vi "re_Edit Remote File.vi"() -> ()   [LabVIEW 2012]
doc: "Edit a remote file by selection and downloading to a temporary file, spawning an editor, and, on completion, uploading the file back to the server when modified. This VI should be run asynchronously so as to allow for multiple editor instances. To do so, open a reference to it with the \"prepare for reentrant run\" option.\n\nBEWARE: since \"System Exec\" is used which calls into C to spawn the editor, each open editor occupies a thread. For this reason this VI has been made part of the \"Other 2\" execution system so that the threads being occupied are unlikely to be used for other tasks. Note though that as a result the number of open remote edit jobs is limited to the number of threads in the \"Other 2\" thread pool, which defaults to 4 under LabVIEW 7 with multithreading enabled."
uses:
  served/ClientSrv Server File Manipulation_srv.ctl
  typedefs/t_ClientSrv Access Levels.ctl
  glb_ClientSrv Globals.vi
panel:
  in  "Case Constant\n(See Context Help)":bool
types:
  T1 = typedef "t_ClientSrv Access Levels.ctl" = enum16{"observer", "operator", "local"}
  T2 = typedef "ClientSrv Server File Manipulation_srv.ctl" = refnum<vi>
  T3 = enum32{"existing file", "new file", "new or existing file", "existing dir", "new dir", "new or existing dir", "existing file (use LLBs)", "new file (use LLBs)", "new or existing file (use LLBs)", "new or existing file or directory (use LLBs)"}
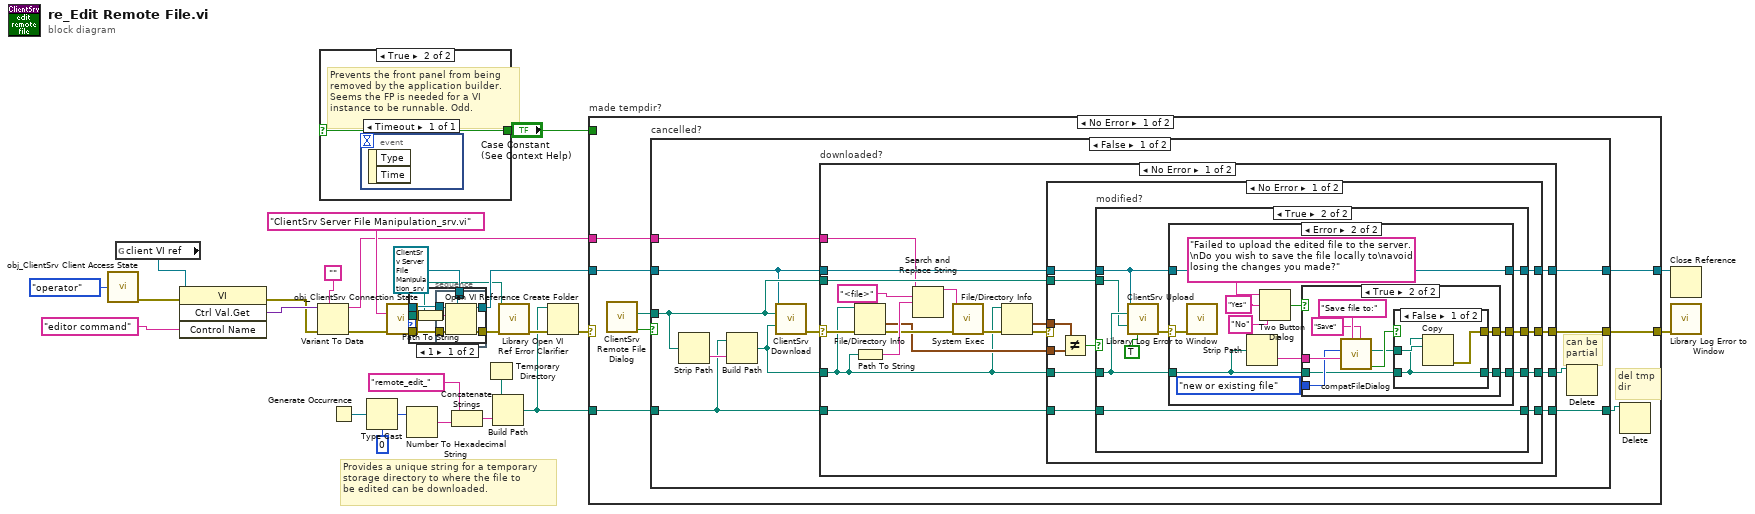
[diagram p0: block diagram]
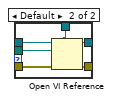
[diagram p2: hidden frame]
diagram:
  # "Provides a unique string for a temporary\nstorage directory to where the file to\nbe edited can be downloaded."
  n1 = call "obj_ClientSrv Client Access State.vi"("access level (observer)"=t_ClientSrv_Access_Levels."operator") -> ("error out"=w9:errorcluster)  [unwired: 13 in, 1 out]
  n2 = global read "glb_ClientSrv Globals.vi" "client VI ref"() -> (w18:refnum<vi>)
  n3 = invoke class="VI" method="Ctrl Val.Get"(reference=w18, error in=w9, "Control Name"="editor command") -> (error out=w14:errorcluster, "Get Control Value Variant"=w16:variant)  [unwired: 1 in, 2 out]
  n4 = Variant To Data(error in=w14, type="", Variant=w16) -> (data=w12:string, error out=w13:errorcluster)
  n5 = case shown="True" "Case Constant\n(See Context Help)" {
    selector: "Case Constant\n(See Context Help)" -> [w31 w32]
    tunnel: [w31 w32] -> w7
    frame False {
    }
    frame True {
      # "Prevents the front panel from being\nremoved by the application builder.\nSeems the FP is needed for a VI\ninstance to be runnable. Odd."
      n6 = event shown="[0] Timeout" {
        selector: _ -> [_]
        dyn-events: _ -> [_]
        timeout: _ -> [_]
        event Timeout {
          n7 = event-data() -> ()  [unwired: 1 in, 2 out]
        }
      }
    }
  }
  n8 = Generate Occurrence() -> (w11:refnum<k4>)
  n9 = Type Cast(type=u32 0, x=w11) -> (*(type *) &x=w29:u32)
  n10 = call "obj_ClientSrv Connection State.vi"("machine{connect}/VI{get state} name (local/no path resolution)"="ClientSrv Server File Manipulation_srv.vi", "error in (no error)"=w13) -> ("server app ref"=w2:refnum<vi>, "resolved server path"=w1:path, "error out"=w3:errorcluster)  [unwired: 6 in, 5 out]
  n11 = Number To Hexadecimal String(2:w29) -> (0:w27:string)  [unwired: 1 in]
  n12 = stacked-sequence {
    tunnel: [w38] -> w4
    tunnel: [w37] -> w6
    tunnel: w3 -> [w36]
    tunnel: w2 -> [w35]
    tunnel: w1 -> [w34]
    tunnel: T2 refnum ("file manipulation") -> [w33]
    frame #0 {
      # "avoid LV8 complaints"
      n13 = Path to Array of Strings(0:w34) -> (2:w39:string[])  [unwired: 1 out]
      n14 = Array Size(array=w39) -> (size(s)=w40:i32)
      n15 = case shown="1" w40 {
        tunnel: w34 -> [w47 w53]
        tunnel: w35 -> [w45 w52]
        tunnel: [w43 w48] -> w38
        tunnel: [w41 w51] -> w37
        tunnel: w33 -> [w42 w50]
        tunnel: w36 -> [w44 w49]
        frame 1 {
          n16 = Path To String(path=w47) -> (string=w46:string)
          n17 = Open VI Reference(type specifier VI Refnum (for type only)=w42, application reference (local)=w45, vi path=w46, error in (no error)=w44) -> (vi reference=w43:T2, error out=w41:errorcluster)  [unwired: 2 in]
        }
        frame Default {
          n18 = Open VI Reference(type specifier VI Refnum (for type only)=w50, application reference (local)=w52, vi path=w53, error in (no error)=w49) -> (vi reference=w48:T2, error out=w51:errorcluster)  [unwired: 2 in]
        }
      }
    }
  }
  n19 = Concatenate Strings("remote_edit_" ("string"), w27) -> (w25:string)
  n20 = Temporary Directory() -> (w24:path)
  n21 = Build Path(base path=w24, name or relative path=w25) -> (appended path=w20:path)
  n22 = call "Library Open VI Ref Error Clarifier.vi"("VI path"=w1, "called VI error (no error)"=w6) -> ("error out"=w23:errorcluster)  [unwired: 13 in]
  n23 = Create Folder(path (use dialog)=w20, error in=w23) -> (error out=w22:errorcluster)  [unwired: 1 in, 2 out]
  n24 = case "made tempdir?" shown="No Error" w22 {
    selector: w22 -> [_ w152]
    tunnel: w4 -> [w61 w153]
    tunnel: [w60 w153] -> w21
    tunnel: w20 -> [w57 _]
    tunnel: [w55 w152] -> w19
    tunnel: w12 -> [w54 _]
    tunnel: w7 -> [_ _]
    frame No Error {
      # "del tmp\ndir"
      n25 = call "ClientSrv Remote File Dialog.vi"() -> ("cancelled"=w59:bool, "path"=w58:path)  [unwired: 10 in]
      n26 = case "cancelled?" shown="False" w59 {
        tunnel: w61 -> [w68 w151]
        tunnel: [w67 w151] -> w60
        tunnel: w58 -> [w69 _]
        tunnel: w57 -> [w66 w150]
        tunnel: [w65 w150] -> w56
        tunnel: [w64 _] -> w55
        tunnel: w54 -> [w62 _]
        frame False {
          # "can be\npartial"
          n27 = Strip Path(path=w69) -> (name=w72:string)  [unwired: 1 out]
          n28 = Build Path(base path=w66, name or relative path=w72) -> (appended path=w70:path)
          n29 = call "ClientSrv Download.vi"("file manipulation"=w68, "remote file"=w69, "local file"=w70) -> ("error out"=w71:errorcluster)  [unwired: 12 in]
          n30 = case "downloaded?" shown="No Error" w71 {
            selector: w71 -> [w87 w147]
            tunnel: w70 -> [w79 w146]
            tunnel: w69 -> [w74 _]
            tunnel: w68 -> [w76 w149]
            tunnel: [w75 w149] -> w67
            tunnel: [w77 w148] -> w65
            tunnel: w66 -> [w82 w148]
            tunnel: [w83 w147] -> w64
            tunnel: [w78 w146] -> w63
            tunnel: w62 -> [w73 _]
            frame No Error {
              n31 = File/Directory Info(path=w79, error in=w87) -> (last mod=w80:timestamp, error out=w86:errorcluster)  [unwired: 5 out]
              n32 = Path To String(path=w79) -> (string=w89:string)
              n33 = Search and Replace String(input string=w73, search string="<file>", replace string=w89) -> (result string=w90:string)  [unwired: 5 in, 3 out]
              n34 = call <vilib>:"System Exec.vi"("error in (no error)"=w86, "command line"=w90) -> ("error out"=w85:errorcluster)  [unwired: 6 in, 3 out]
              n35 = File/Directory Info(path=w79, error in=w85) -> (last mod=w81:timestamp, error out=w84:errorcluster)  [unwired: 5 out]
              n36 = case shown="No Error" w84 {
                selector: w84 -> [_ w144]
                tunnel: [w92 w144] -> w83
                tunnel: w82 -> [w97 w142]
                tunnel: w81 -> [w101 _]
                tunnel: w80 -> [w100 _]
                tunnel: w79 -> [w98 w143]
                tunnel: [w96 w143] -> w78
                tunnel: [w95 w142] -> w77
                tunnel: w76 -> [w94 w145]
                tunnel: [w93 w145] -> w75
                tunnel: w74 -> [w91 _]
                frame No Error {
                  n37 = Not Equal?(x=w101, y=w100) -> (x != y?=w99:bool)
                  n38 = case "modified?" shown="True" w99 {
                    tunnel: w98 -> [w104 w110]
                    tunnel: w97 -> [w103 w113]
                    tunnel: [w104 w107] -> w96
                    tunnel: [w103 w113] -> w95
                    tunnel: w94 -> [w102 w109]
                    tunnel: [w102 w108] -> w93
                    tunnel: [_ w111] -> w92
                    tunnel: w91 -> [_ w106]
                    frame False {
                    }
                    frame True {
                      n39 = call "ClientSrv Upload.vi"("file manipulation"=w109, "local file"=w110, "remote file"=w106, "overwrite (F)"=TRUE) -> ("error out"=w112:errorcluster)  [unwired: 11 in]
                      n40 = case shown="Error" w112 {
                        selector: w112 -> [w116 w125]
                        tunnel: [w116 w117] -> w111
                        tunnel: w110 -> [w114 w121]
                        tunnel: w109 -> [w115 w126]
                        tunnel: [w115 w126] -> w108
                        tunnel: [w114 w119] -> w107
                        frame No Error {
                        }
                        frame Error {
                          n41 = call "Library Log Error to Window.vi"("error in (no error)"=w125) -> ()  [unwired: 13 in, 2 out]
                          n42 = Strip Path(path=w121) -> (name=w120:string)  [unwired: 1 out]
                          n43 = Two Button Dialog(message="Failed to upload the edited file to the server.\nDo you wish to save the file locally to\navoid losing the changes you made?", 1:"No" ("F button name (\"Cancel\")"), 2:"Yes" ("T button name (\"OK\")")) -> (T button?=w122:bool)
                          n44 = case shown="True" w122 {
                            tunnel: w121 -> [w128 w131]
                            tunnel: w120 -> [_ w136]
                            tunnel: [w128 w130] -> w119
                            tunnel: T3."new or existing file" ("select mode (2)") -> [_ w133]
                            tunnel: [_ w129] -> w117
                            frame False {
                            }
                            frame True {
                              n45 = call <vilib>:"compatFileDialog.vi"("button label"="Save", "prompt"="Save file to:", "default name"=w136, "select mode (2)"=w133) -> ("cancelled"=w134:bool, "path"=w132:path)  [unwired: 5 in, 1 out]
                              n46 = case shown="False" w134 {
                                tunnel: w132 -> [w140 _]
                                tunnel: w131 -> [w139 w141]
                                tunnel: [w139 w141] -> w130
                                tunnel: [w138 _] -> w129
                                frame False {
                                n47 = Copy(10:w140, 11:w139) -> (0:w138:errorcluster)  [unwired: 3 in, 2 out]
                                }
                                frame True {
                                }
                              }
                            }
                          }
                        }
                      }
                    }
                  }
                }
                frame Error {
                }
              }
            }
            frame Error {
            }
          }
          n48 = Delete(path (use dialog)=w63) -> ()  [unwired: 4 in, 3 out]
        }
        frame True {
        }
      }
      n49 = Delete(path (use dialog)=w56) -> ()  [unwired: 4 in, 3 out]
    }
    frame Error {
    }
  }
  n50 = Close Reference(reference=w21) -> ()  [unwired: 1 in, 1 out]
  n51 = call "Library Log Error to Window.vi"("error in (no error)"=w19) -> ()  [unwired: 13 in, 2 out]
